vi "Updates.vi"(8 "error in (no error)":errorcluster, 10 "Readings in":T1, 11 "VISA Refnum in":refnum<visa-resource-name>) -> (0 "error out":errorcluster, 2 "Readings out":T1, 3 "VISA Refnum out":refnum<visa-resource-name>)   [LabVIEW 2022 SP3]
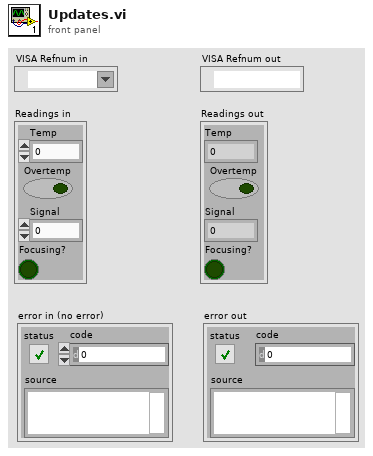
[diagram p1: front panel]
types:
  T1 = cluster{"Temp":dbl, "Overtemp":bool, "Signal":u8, "Focusing?":bool}
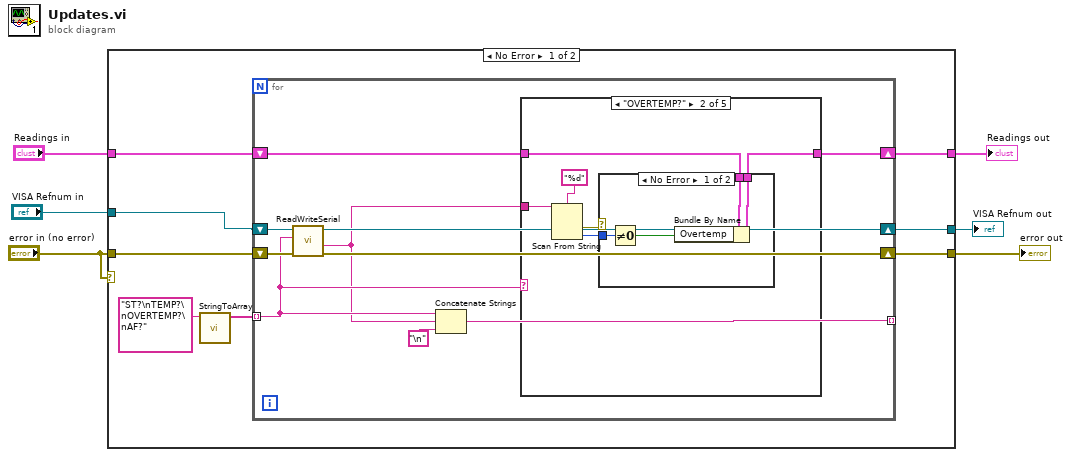
[diagram p0: block diagram]
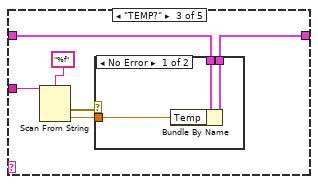
[diagram p4: hidden frame]
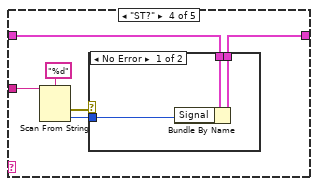
[diagram p6: hidden frame]
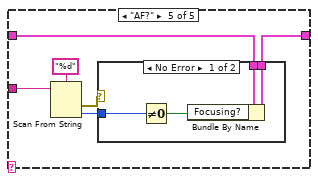
[diagram p8: hidden frame]
diagram:
  n1 = case shown="No Error" "error in (no error)" {
    tunnel: [w14 w70] -> w6
    tunnel: [w13 w68] -> w5
    tunnel: [w12 w69] -> w4
    tunnel: "error in (no error)" -> [w11 w68]
    tunnel: "VISA Refnum in" -> [w10 w69]
    tunnel: "Readings in" -> [w9 w70]
    frame No Error {
      n2 = call "StringToArray.vi"("write buffer"="ST?\nTEMP?\nOVERTEMP?\nAF?") -> ("Array"=w7:string[])  [unwired: 10 in]
      n3 = for {
        tunnel: w7 -> [w18] mode=indexing
        shift-right: [w24] -> w13
        shift-left: w11 -> [w22]
        shift-right: [w23] -> w12
        shift-left: w10 -> [w21]
        tunnel: [w20] -> _ mode=indexing
        shift-right: [w15] -> w14
        shift-left: w9 -> [w16]
        n4 = call "ReadWriteSerial.vi"("error in (no error)"=w22, "cmd"=w18, "VISA Refnum in"=w21) -> ("error out"=w24:errorcluster, "Reply"=w17:string, "VISA Refnum out"=w23:refnum<visa-resource-name>)  [unwired: 5 in, 1 out]
        n5 = Concatenate Strings(w18, w17, "\n" ("regular expression")) -> (w20:string)
        n6 = case shown="\"OVERTEMP?\"" w18 {
          tunnel: w17 -> [_ w31 w42 w52 w60]
          tunnel: w16 -> [w25 w28 w40 w49 w59]
          tunnel: [w25 w27 w38 w48 w58] -> w15
          frame Default {
          }
          frame "OVERTEMP?" {
            n7 = Scan From String(format string="%d", input string=w31) -> (error out=w26:errorcluster, output 1=w29:i32)  [unwired: 3 in, 2 out]
            n8 = case shown="No Error" w26 {
              tunnel: w29 -> [w35 _]
              tunnel: w28 -> [w34 w36]
              tunnel: [w33 w36] -> w27
              frame No Error {
                n9 = Not Equal To 0?(x=w35) -> (x != 0?=w32:bool)
                n10 = Bundle By Name(cluster=w34, "Overtemp"=w32) -> (w33:T1)
              }
              frame Error {
              }
            }
          }
          frame "TEMP?" {
            n11 = Scan From String(format string="%f", input string=w42) -> (error out=w37:errorcluster, output 1=w39:dbl)  [unwired: 3 in, 2 out]
            n12 = case shown="No Error" w37 {
              tunnel: w40 -> [w45 w46]
              tunnel: w39 -> [w44 _]
              tunnel: [w43 w46] -> w38
              frame No Error {
                n13 = Bundle By Name(cluster=w45, "Temp"=w44) -> (w43:T1)
              }
              frame Error {
              }
            }
          }
          frame "ST?" {
            n14 = Scan From String(format string="%d", input string=w52) -> (error out=w47:errorcluster, output 1=w50:i32)  [unwired: 3 in, 2 out]
            n15 = case shown="No Error" w47 {
              tunnel: w50 -> [w55 _]
              tunnel: w49 -> [w54 w56]
              tunnel: [w53 w56] -> w48
              frame No Error {
                n16 = Bundle By Name(cluster=w54, "Signal"=w55) -> (w53:T1)
              }
              frame Error {
              }
            }
          }
          frame "AF?" {
            n17 = Scan From String(format string="%d", input string=w60) -> (error out=w57:errorcluster, output 1=w61:i32)  [unwired: 3 in, 2 out]
            n18 = case shown="No Error" w57 {
              tunnel: w61 -> [w66 _]
              tunnel: w59 -> [w64 w67]
              tunnel: [w63 w67] -> w58
              frame No Error {
                n19 = Not Equal To 0?(x=w66) -> (x != 0?=w65:bool)
                n20 = Bundle By Name(cluster=w64, "Focusing?"=w65) -> (w63:T1)
              }
              frame Error {
              }
            }
          }
        }
      }
    }
    frame Error {
    }
  }
  "Readings out" <- w6
  "error out" <- w5
  "VISA Refnum out" <- w4
